vi "TS20170120_0749_V1_Kalibrierung.vi"() -> ()   [LabVIEW 2018]
uses:
  <vilib>/gmath/NI_Gmath.lvlib
  <vilib>/Analysis/NI_AALBase.lvlib
panel:
  in  "Optionsauswahl 2":bool
  in  "Optionsfelder 2":T1(radio)
  in  "Messen":bool
  in  "Kalibrieren":bool
  in  "Bref_5/mT":dbl=75.0
  in  "Bref_4/mT":dbl=60.0
  in  "Bref_3/mT":dbl=45.0
  in  "Bref_2/mT":dbl=30.0
  in  "Bref_1/mT":dbl=15.0
  in  "Reset_Bref5":bool
  in  "Reset_Bref4":bool
  in  "Reset_Bref3":bool
  in  "Reset_Bref2":bool
  in  "Reset_Bref1":bool
  out "Median":dbl[](array[numeric])
  in  "Umess_in / mV":dbl
  in  "Anwendung beenden":bool
  out "Bmess / mT":dbl
  in  "obere Grenze Bref/mT":dbl=100.0
  in  "untere Grenze Bref/mT":dbl
  in  "Anzahl Punkte":i32=1024
  out "Messwerte\nUmess,ref / mV":dbl[][](array[numeric])
  in  "Interpolationstyp":i32(ring)=1 items=["Nächste", "Linear", "Spline", "Hermite", "Lagrange"]
  out "Darstellung der Funktion":cluster{"xi used":dbl[], "yi":dbl[]}[](graph)
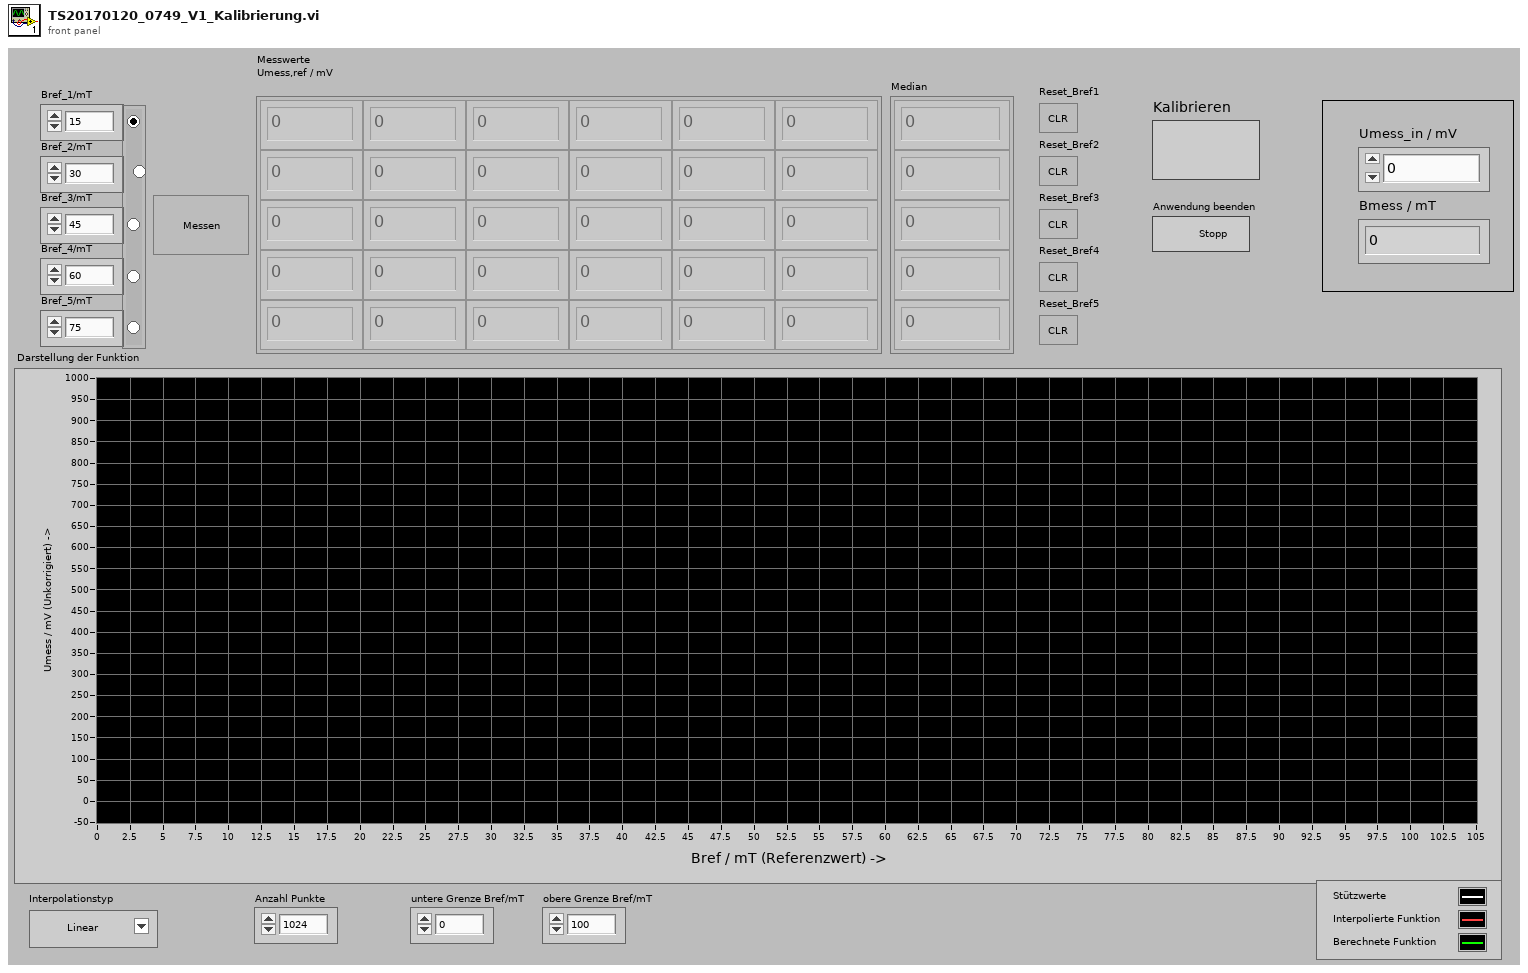
[diagram p1: front panel]
types:
  T1 = enum32{"Optionsauswahl 1", "Optionsauswahl 3", "Optionsauswahl 4", "Optionsauswahl 5"}
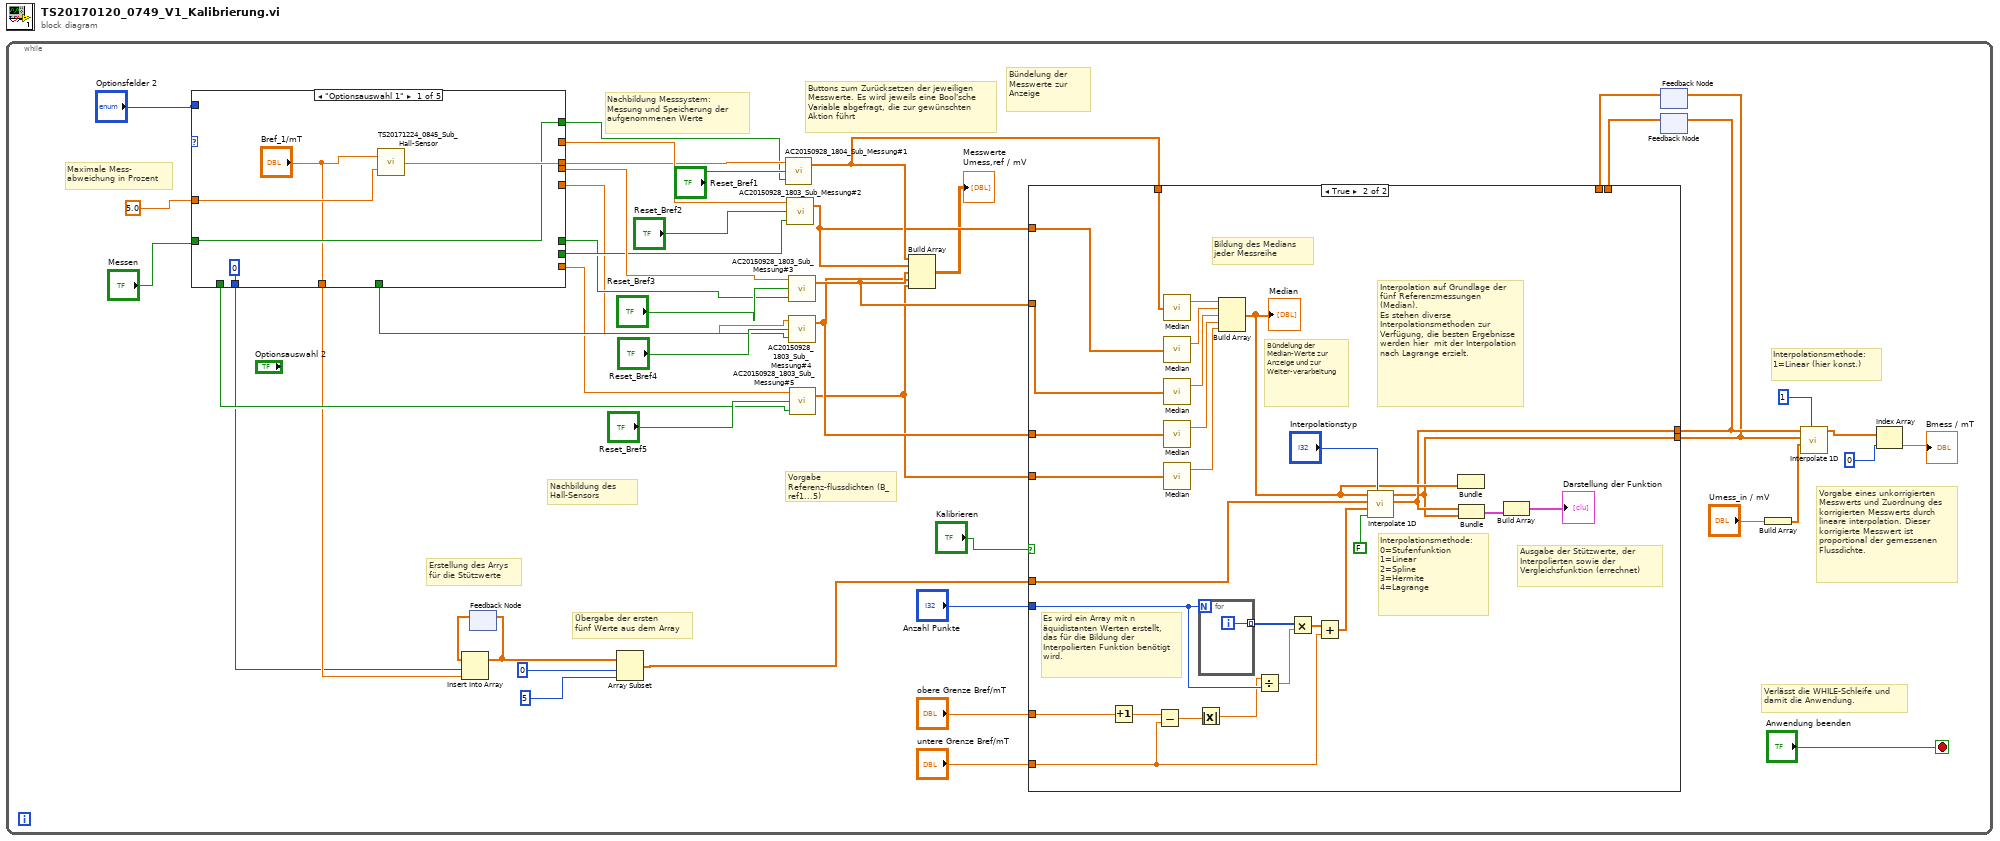
[diagram p0: block diagram]
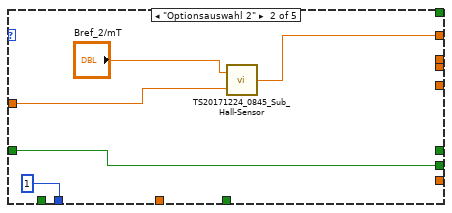
[diagram p2: hidden frame]
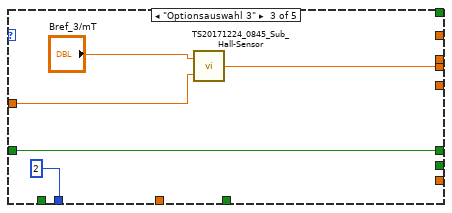
[diagram p3: hidden frame]
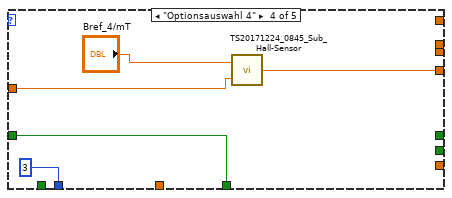
[diagram p4: hidden frame]
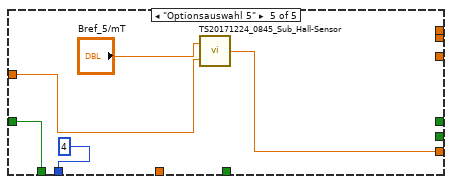
[diagram p5: hidden frame]
diagram:
  n1 = while {
    stop <- "Anwendung beenden" stop-if-true
    # "Erstellung des Arrys \nfür die Stützwerte"
    # "Übergabe der ersten \nfünf Werte aus dem Array"
    # "Maximale Mess-\nabweichung in Prozent"
    # "Vorgabe eines unkorrigierten Messwerts und Zuordnung des korrigierten Messwerts durch lineare interpolation. Dieser korrigierte Messwert ist proportional der gemessenen Flussdichte."
    # "Verlässt die WHILE-Schleife und damit die Anwendung."
    # "Interpolationsmethode:\n1=Linear (hier konst.)"
    # "Buttons zum Zurücksetzen der jeweiligen Messwerte. Es wird jeweils eine Bool'sche Variable abgefragt, die zur gewünschten Aktion führt"
    # "Bündelung der Messwerte zur Anzeige"
    # "Nachbildung Messsystem:\nMessung und Speicherung der aufgenommenen Werte"
    # "Nachbildung des \nHall-Sensors"
    # "Vorgabe Referenz-flussdichten (B_ref1...5)"
    n2 = case shown="\"Optionsauswahl 1\"" {
      selector: _ -> [_ _ _ _ _]
      tunnel: 5.0 -> [w51 w55 w60 w66 w70]
      tunnel: [_ _ _ _ w69] -> w15
      tunnel: [_ _ _ w64 _] -> w16
      tunnel: [_ _ w59 _ _] -> w26
      tunnel: [_ w54 _ _ _] -> w30
      tunnel: [w50 _ _ _ _] -> w29
      tunnel: "Messen" -> [w49 w53 w58 w63 w68]
      tunnel: [w49 _ _ _ _] -> w21
      tunnel: [_ w53 _ _ _] -> w20
      tunnel: [_ _ w58 _ _] -> w19
      tunnel: [_ _ _ w63 _] -> w18
      tunnel: [_ _ _ _ w68] -> w17
      tunnel: "Optionsfelder 2" -> [_ _ _ _ _]
      tunnel: ["Bref_1/mT" _ _ _ _] -> w8
      tunnel: [0 1 2 3 4] -> w2
      frame "Optionsauswahl 1" {
        n3 = call "TS20171224_0845_Sub_Hall-Sensor.vi"("Max_Abweichung\n(% vom richtigen Wert)"=w51, "Referenzflussdichte\nB_ref_in"="Bref_1/mT") -> ("Messspannung\nU_mess_out"=w50:dbl)
      }
      frame "Optionsauswahl 2" {
        n4 = call "TS20171224_0845_Sub_Hall-Sensor.vi"("Max_Abweichung\n(% vom richtigen Wert)"=w55, "Referenzflussdichte\nB_ref_in"="Bref_2/mT") -> ("Messspannung\nU_mess_out"=w54:dbl)
      }
      frame "Optionsauswahl 3" {
        n5 = call "TS20171224_0845_Sub_Hall-Sensor.vi"("Max_Abweichung\n(% vom richtigen Wert)"=w60, "Referenzflussdichte\nB_ref_in"="Bref_3/mT") -> ("Messspannung\nU_mess_out"=w59:dbl)
      }
      frame "Optionsauswahl 4" {
        n6 = call "TS20171224_0845_Sub_Hall-Sensor.vi"("Max_Abweichung\n(% vom richtigen Wert)"=w66, "Referenzflussdichte\nB_ref_in"="Bref_4/mT") -> ("Messspannung\nU_mess_out"=w64:dbl)
      }
      frame "Optionsauswahl 5" {
        n7 = call "TS20171224_0845_Sub_Hall-Sensor.vi"("Max_Abweichung\n(% vom richtigen Wert)"=w70, "Referenzflussdichte\nB_ref_in"="Bref_5/mT") -> ("Messspannung\nU_mess_out"=w69:dbl)
      }
    }
    n8 = feedback #1() -> (w7:dbl[])  [unwired: 1 in]
    n9 = Insert Into Array(array=w7, index=w2, new element=w8) -> (w6:dbl[])
    n10 = feedback-in #1(w6) -> ()
    n11 = Array Subset(array=w6, index=0, length=5) -> (w3:dbl[])
    n12 = call "AC20150928_1804_Sub_Messung#1.vi"("Reset"=w21, "Übernehmen"="Reset_Bref1", "U_mess_in"=w29) -> ("Mess_Array_Out[6]"=w14:dbl[])  [unwired: 1 in]
    n13 = call "AC20150928_1803_Sub_Messung#2.vi"("Reset"=w20, "Übernehmen"="Reset_Bref2", "U_mess_in"=w30) -> ("Mess_Array_Out[6]"=w13:dbl[])  [unwired: 1 in]
    n14 = call "AC20150928_1803_Sub_Messung#3.vi"("Reset"=w19, "Übernehmen"="Reset_Bref3", "U_mess_in"=w26) -> ("Mess_Array_Out[6]"=w12:dbl[])  [unwired: 1 in]
    n15 = call "AC20150928_1803_Sub_Messung#4.vi"("Reset"=w18, "Übernehmen"="Reset_Bref4", "U_mess_in"=w16) -> ("Mess_Array_Out[6]"=w11:dbl[])  [unwired: 1 in]
    n16 = call "AC20150928_1803_Sub_Messung#5.vi"("Reset"=w17, "Übernehmen"="Reset_Bref5", "U_mess_in"=w15) -> ("Mess_Array_Out[6]"=w10:dbl[])  [unwired: 1 in]
    n17 = Build Array(w14, w13, w12, w11, w10) -> (→"Messwerte\nUmess,ref / mV":dbl[][])
    n18 = feedback #2() -> (w32:dbl[])  [unwired: 1 in]
    n19 = feedback #3() -> (w34:dbl[])  [unwired: 1 in]
    n20 = case shown="True" "Kalibrieren" {
      tunnel: "untere Grenze Bref/mT" -> [_ w101]
      tunnel: "Anzahl Punkte" -> [_ w100]
      tunnel: "obere Grenze Bref/mT" -> [_ w99]
      tunnel: [w72 w80] -> w33
      tunnel: [w73 w81] -> w35
      tunnel: w34 -> [w73 _]
      tunnel: w32 -> [w72 _]
      tunnel: w14 -> [_ w79]
      tunnel: w13 -> [_ w78]
      tunnel: w12 -> [_ w77]
      tunnel: w11 -> [_ w76]
      tunnel: w10 -> [_ w75]
      tunnel: w3 -> [_ w74]
      frame False {
      }
      frame True {
        # "Bildung des Medians\njeder Messreihe"
        # "Bündelung der Median-Werte zur Anzeige und zur Weiter-verarbeitung"
        # "Interpolationsmethode:\n0=Stufenfunktion\n1=Linear\n2=Spline\n3=Hermite\n4=Lagrange"
        # "Ausgabe der Stützwerte, der Interpolierten sowie der Vergleichsfunktion (errechnet)"
        # "Interpolation auf Grundlage der fünf Referenzmessungen (Median).\nEs stehen diverse Interpolationsmethoden zur Verfügung, die besten Ergebnisse werden hier  mit der Interpolation nach Lagrange erzielt."
        # "Es wird ein Array mit n äquidistanten Werten erstellt, das für die Bildung der Interpolierten Funktion benötigt wird."
        n21 = Increment(x=w99) -> (x+1=w89:dbl)
        n22 = Subtract(x=w89, y=w101) -> (x-y=w94:dbl)
        n23 = call <vilib>:"Median.vi"("X"=w79) -> ("median"=w87:dbl)  [unwired: 1 out]
        n24 = call <vilib>:"Median.vi"("X"=w78) -> ("median"=w86:dbl)  [unwired: 1 out]
        n25 = call <vilib>:"Median.vi"("X"=w77) -> ("median"=w85:dbl)  [unwired: 1 out]
        n26 = call <vilib>:"Median.vi"("X"=w76) -> ("median"=w84:dbl)  [unwired: 1 out]
        n27 = call <vilib>:"Median.vi"("X"=w75) -> ("median"=w83:dbl)  [unwired: 1 out]
        n28 = Absolute Value(x=w94) -> (abs(x)=w90:dbl)
        n29 = for {
          N: w100 -> [_]
          tunnel: [w102] -> w93 mode=indexing
          i -> [w102]
        }
        n30 = Build Array(w87, w86, w85, w84, w83) -> (w82:dbl[])
        "Median" <- w82
        n31 = Divide(x=w90, y=w100) -> (x/y=w92:dbl)
        n32 = Multiply(x=w93, y=w92) -> (x*y=w91:dbl[])
        n33 = Add(x=w91, y=w101) -> (x+y=w88:dbl[])
        n34 = call <vilib>:"Interpolate 1D.vi"("method"="Interpolationstyp", "X is monotonic"=FALSE, "xi"=w88, "X"=w74, "Y"=w82) -> ("xi used"=w81:dbl[], "yi"=w80:dbl[])  [unwired: 4 in, 1 out]
        n35 = Bundle(w82) -> ()  [unwired: 2 in, 1 out]
        n36 = Bundle("xi used"=w81, "yi"=w80) -> (w96:cluster{"xi used":dbl[], "yi":dbl[]})  [unwired: 1 in]
        n37 = Build Array(w96) -> (→"Darstellung der Funktion":cluster{"xi used":dbl[], "yi":dbl[]}[])  [unwired: 1 in]
      }
    }
    n38 = feedback-in #2(w33) -> ()
    n39 = feedback-in #3(w35) -> ()
    n40 = Build Array("Umess_in / mV") -> (w41:dbl[])
    n41 = call <vilib>:"Interpolate 1D.vi"("method"=1, "xi"=w41, "X"=w33, "Y"=w35) -> ("yi"=w39:dbl[])  [unwired: 5 in, 2 out]
    n42 = Index Array(array=w39, index=0) -> (element=→"Bmess / mT":dbl)
  }
